vi "Get stimulus stat.vi"(9 "stimphases":T1, 10 "time":dbl, 11 "Stimulus":T2={"type"=enum."Zero", "sinfreq start"=0.0, "sinfreq end"=0.0, "sinamp start"=0.0, "sinamp end"=0.0, "noise freq lo"=0.0, "noise freq hi"=0.0, "noiseamp start"=0.0, "noiseamp end"=0.0, "stimdur"=0.0, "before dur"=0.0, "after dur"=0.0, "pulse data"={"time"=[], "phase/vel"=[], "dir/shift"=[], "amplitude"=[], "duration"=[]}} {"noise freq hi" min=0.0 step=0.5; "noise freq lo" min=0.0 step=0.5; "noiseamp end" min=0.0 step=0.5; "noiseamp start" min=0.0 step=0.5}) -> (1 "noiseamp":dbl, 2 "sinamp":dbl, 3 "sinfreq":dbl)   [LabVIEW 2013]
uses:
  Stimulus.ctl
  Stimulus type.ctl
  Pulse data.ctl
  Stim phases.ctl
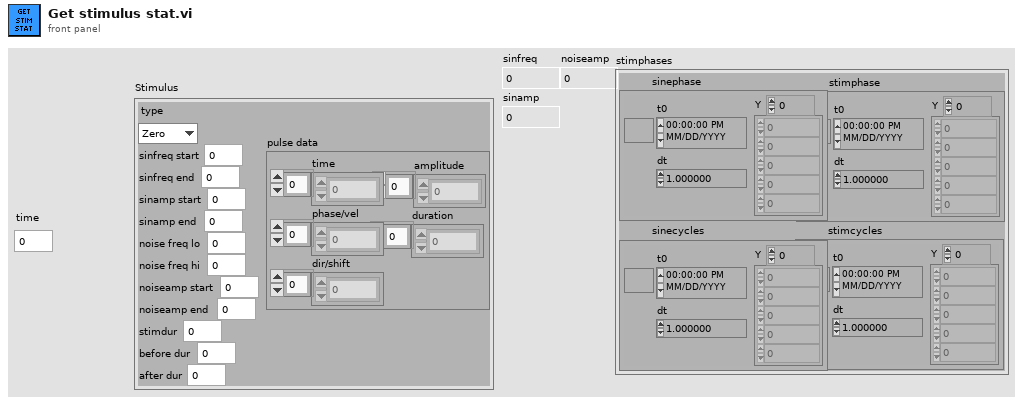
[diagram p1: front panel]
types:
  T1 = typedef "Stim phases.ctl" = cluster{"sinephase":waveform(dbl), "sinecycles":waveform(dbl), "stimphase":waveform(dbl), "stimcycles":waveform(dbl)}
  T2 = typedef "Stimulus.ctl" = cluster{"type":T3, "sinfreq start":dbl, "sinfreq end":dbl, "sinamp start":dbl, "sinamp end":dbl, "noise freq lo":dbl, "noise freq hi":dbl, "noiseamp start":dbl, "noiseamp end":dbl, "stimdur":dbl, "before dur":dbl, "after dur":dbl, "pulse data":T4}
  T3 = typedef "Stimulus type.ctl" = enum16{"Sine", "Zero", "Frequency sweep", "Two frequency", "Amplitude sweep", "Pulses", "Shifts", "Ramps"}
  T4 = typedef "Pulse data.ctl" = cluster{"time":dbl[], "phase/vel":dbl[], "dir/shift":dbl[], "amplitude":dbl[], "duration":dbl[]}
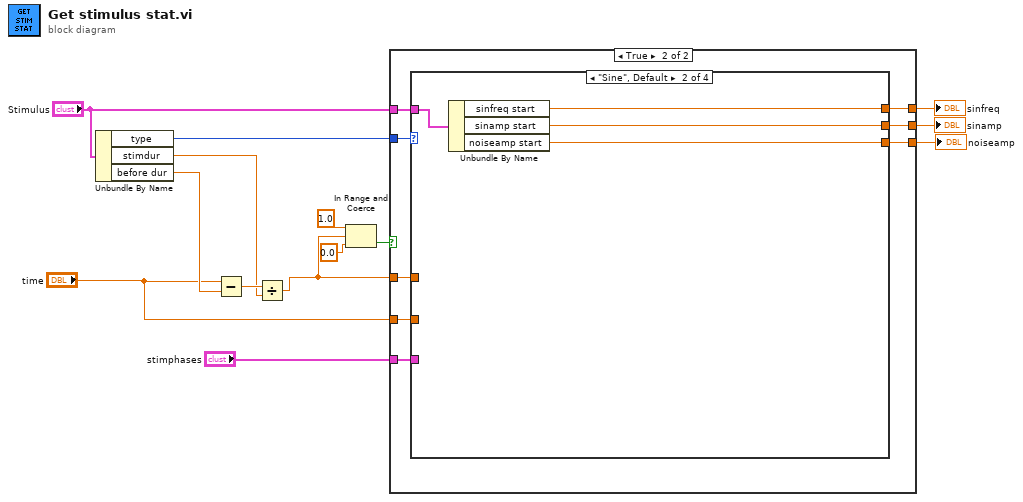
[diagram p0: block diagram]
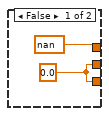
[diagram p2: hidden frame]
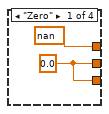
[diagram p3: hidden frame]
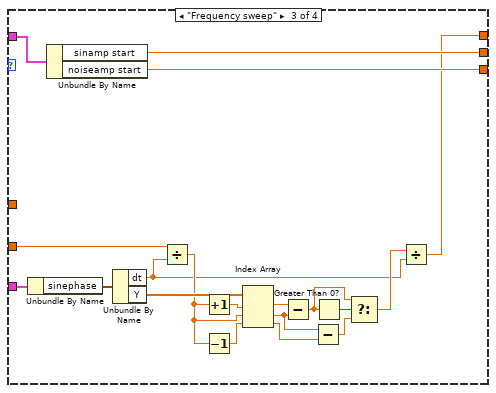
[diagram p4: hidden frame]
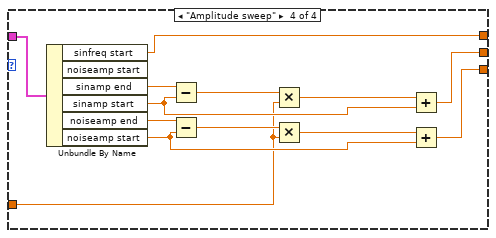
[diagram p5: hidden frame]
diagram:
  n1 = Unbundle By Name("Stimulus") -> ("type"=w14:T3, "stimdur"=w7:dbl, "before dur"=w8:dbl)
  n2 = Subtract(x="time", y=w8) -> (x-y=w9:dbl)
  n3 = Divide(x=w9, y=w7) -> (x/y=w6:dbl)
  n4 = In Range and Coerce(upper limit=1.0, x=w6, lower limit=0.0) -> (In Range?=w3:bool)  [unwired: 1 out]
  n5 = case shown="True" w3 {
    tunnel: w14 -> [_ w24]
    tunnel: "Stimulus" -> [_ w23]
    tunnel: [nan ("sinfreq start") w22] -> w12
    tunnel: [w15 w21] -> w11
    tunnel: [w15 w20] -> w10
    tunnel: w6 -> [_ w19]
    tunnel: "stimphases" -> [_ w18]
    tunnel: "time" -> [_ w17]
    frame False {
      w15 = 0.0 ("sinamp start")
    }
    frame True {
      n6 = case shown="\"Sine\", Default" w24 {
        tunnel: w23 -> [_ w30 w49 w62]
        tunnel: [nan ("sinfreq start") w29 w31 w57] -> w22
        tunnel: [w25 w28 w48 w52] -> w21
        tunnel: [w25 w27 w47 w51] -> w20
        tunnel: w19 -> [_ _ _ w50]
        tunnel: w18 -> [_ _ w46 _]
        tunnel: w17 -> [_ _ w44 _]
        frame "Zero" {
          w25 = 0.0 ("sinamp start")
        }
        frame "Sine", Default {
          n7 = Unbundle By Name(w30) -> ("sinfreq start"=w29:dbl, "sinamp start"=w28:dbl, "noiseamp start"=w27:dbl)
        }
        frame "Frequency sweep" {
          n8 = Unbundle By Name(w46) -> ("sinephase"=w45:waveform(dbl))
          n9 = Unbundle By Name(w49) -> ("sinamp start"=w48:dbl, "noiseamp start"=w47:dbl)
          n10 = Unbundle By Name(w45) -> ("dt"=w32:dbl, "Y"=w43:dbl[])
          n11 = Divide(x=w44, y=w32) -> (x/y=w41:dbl)
          n12 = Increment(x=w41) -> (x+1=w42:dbl)
          n13 = Decrement(x=w41) -> (x-1=w40:dbl)
          n14 = Index Array(array=w43, index #1=w42, index #2=w41, index #3=w40) -> (element #1=w39:dbl, element #2=w38:dbl, element #3=w37:dbl)
          n15 = Subtract(x=w39, y=w38) -> (x-y=w35:dbl)
          n16 = Subtract(x=w38, y=w37) -> (x-y=w34:dbl)
          n17 = Greater Than 0?(x=w35) -> (x > 0?=w36:bool)
          n18 = Select(t=w35, s=w36, f=w34) -> (s? t:f=w33:dbl)
          n19 = Divide(x=w33, y=w32) -> (x/y=w31:dbl)
        }
        frame "Amplitude sweep" {
          n20 = Unbundle By Name(w62) -> ("sinfreq start"=w57:dbl, "sinamp end"=w61:dbl, "sinamp start"=w58:dbl, "noiseamp end"=w54:dbl, "noiseamp start"=w53:dbl)  [unwired: 1 out]
          n21 = Subtract(x=w61, y=w58) -> (x-y=w60:dbl)
          n22 = Subtract(x=w54, y=w53) -> (x-y=w55:dbl)
          n23 = Multiply(x=w60, y=w50) -> (x*y=w59:dbl)
          n24 = Multiply(x=w55, y=w50) -> (x*y=w56:dbl)
          n25 = Add(x=w59, y=w58) -> (x+y=w52:dbl)
          n26 = Add(x=w56, y=w53) -> (x+y=w51:dbl)
        }
      }
    }
  }
  "sinfreq" <- w12
  "sinamp" <- w11
  "noiseamp" <- w10
